vi "Bundle.vi"(4 "Success?":bool, 6 "Calibration Needed?":bool, 7 "Hours since last Cal":dbl, 8 "error in (no error)":errorcluster, 9 "Current T":dbl, 10 "Last Cal T":dbl, 11 "NI DMM Calibration Data in":refnum<class "NI DMM Calibration Data.lvclass">) -> (0 "error out":errorcluster, 3 "NI DMM Calibration Data out":refnum<class "NI DMM Calibration Data.lvclass">)   [LabVIEW 2020, in "NI DMM Driver.lvlib" / "NI DMM Calibration Data.lvclass"]
doc: "Populate the class. \nDoes not set the values set by Initialize."
uses:
  NI DMM Calibration Data.lvclass
  NI DMM Calibration Data.lvclass/NI DMM Calibration Data.ctl
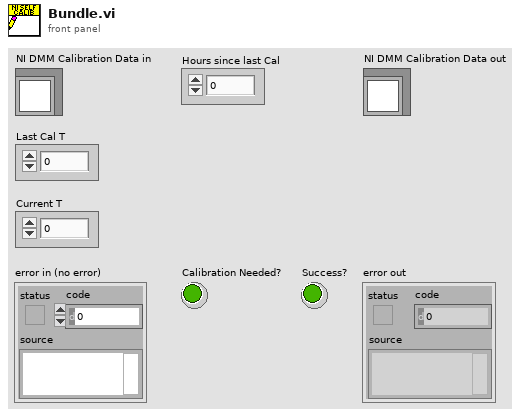
[diagram p1: front panel]
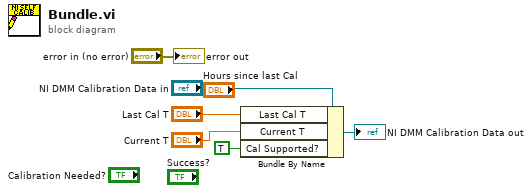
[diagram p0: block diagram]
diagram:
  n1 = Bundle By Name(cluster="NI DMM Calibration Data in", "Last Cal T"="Last Cal T", "Current T"="Current T", "Cal Supported?"=TRUE) -> (→"NI DMM Calibration Data out":refnum<class "NI DMM Calibration Data.lvclass">)
  "error out" <- "error in (no error)"
